vi "Find Class by Name.vi"(8 "error in (no error)":errorcluster, 10 "Name":string, 11 "Installed Instruments":refnum<class "Instrument.lvclass">[](array[class])) -> (0 "error out":errorcluster, 2 "Found?":bool, 3 "Instrument out":refnum<class "Instrument.lvclass">)   [LabVIEW 2019, in "Control Experiment.lvclass"]
uses:
  Control Experiment.lvclass
  <userlib>/LevyLab/Instrument Framework/Instrument/Instrument.lvclass
  C:/Program Files/National Instruments/LabVIEW 2019/vi.lib/JKI/JKI SMO/SMO/SMO.lvclass
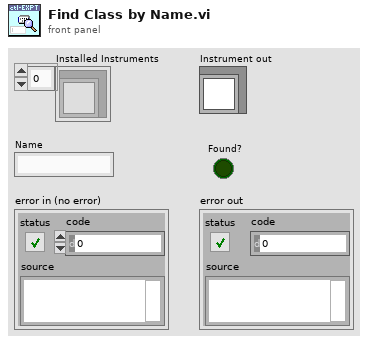
[diagram p1: front panel]
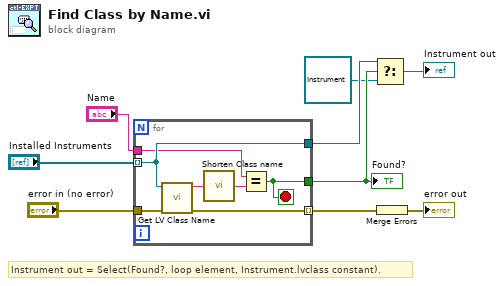
[diagram p0: block diagram]
diagram:
  # "Instrument out = Select(Found?, loop element, Instrument.lvclass constant)."
  n1 = for {
    tunnel: "Installed Instruments" -> [w16] mode=indexing
    tunnel: "Name" -> [w10]
    tunnel: [w16] -> w2
    tunnel: "error in (no error)" -> [w14]
    tunnel: [w15] -> w8 mode=indexing
    tunnel: [w12] -> w4
    stop <- w12 stop-if-true
    n2 = call <vilib>:"Get LV Class Name.vi"("error in (no error)"=w14, "object"=w16) -> ("error out"=w15:errorcluster, "class name"=w13:string)  [unwired: 8 in]
    n3 = call "Shorten Class name.vi"("Qualified Class Name"=w13) -> ("Name"=w11:string)
    n4 = Equal?(x=w10, y=w11) -> (x = y?=w12:bool)
  }
  "Found?" <- w4
  n5 = Select(t=w2, s=w4, f=refnum<class "Instrument.lvclass"> refnum) -> (s? t:f=→"Instrument out":refnum<class "Instrument.lvclass">)
  n6 = Merge Errors(w8) -> (→"error out":errorcluster)
